vi "$UTIL_Timer.vi"(8 "Auto Reset":bool=TRUE, 9 "Reset":bool, 10 "Time (sec)":dbl=3.0, 11 "Start":bool) -> (0 "Timed Out":bool, 1 "Running":bool, 2 "Numeric 2":dbl, 3 "Elapsed":dbl, 4 "TO Trig":bool, 5 "Is Reset?":bool)   [LabVIEW 2024]
doc: "Uses the second timer to determind when Time (sec) have passed when Start is TRUE. The actual time passes is captured in Lap (sec) \nAutoReset is enabled by default. When enabled, at time out, the values is captured, and the TimeOut set to TRUE for one loop then both are RESET. When not enabled, then a RESET command or another START command are requied to reset both the value and TimeOut Flag.\n\n(The functionality could be expanded to measure elapse time on Mark.)"
panel:
  in  "Init":bool
  out "Boolean":bool=TRUE
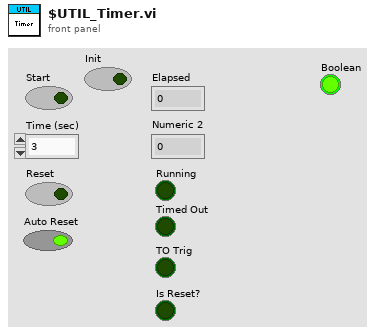
[diagram p1: front panel]
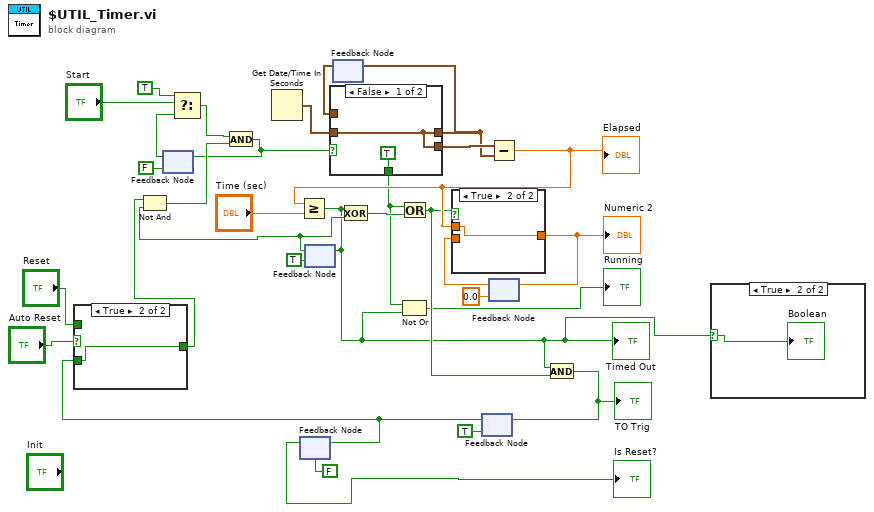
[diagram p0: block diagram]
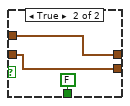
[diagram p5: hidden frame]
diagram:
  n1 = feedback #1(FALSE) -> (w18:bool)
  n2 = Select(t=TRUE, s="Start", f=w18) -> (s? t:f=w16:bool)
  n3 = Get Date/Time In Seconds() -> (seconds since 1Jan1904=w21:timestamp)
  n4 = feedback #2(FALSE) -> (→"Is Reset?":bool)
  n5 = feedback #3(TRUE) -> (w15:bool)
  n6 = feedback #4() -> (w22:timestamp)  [unwired: 1 in]
  n7 = feedback #5(TRUE) -> (w3:bool)
  n8 = case shown="True" "Auto Reset" {
    tunnel: "Reset" -> [w32 _]
    tunnel: [w32 w33] -> w12
    tunnel: w3 -> [_ w33]
    frame False {
    }
    frame True {
    }
  }
  n9 = Not And(1:w15, 2:w12) -> (0:w6:bool)
  n10 = And(x=w16, y=w6) -> (x .and. y?=w4:bool)
  n11 = feedback-in #1(w4) -> ()
  n12 = feedback-in #2(w3) -> ()
  n13 = case shown="False" w4 {
    tunnel: w21 -> [w35 w37]
    tunnel: [w35 w38] -> w23
    tunnel: w22 -> [_ w38]
    tunnel: [w35 w37] -> w24
    tunnel: [TRUE FALSE] -> w8
    frame False {
    }
    frame True {
    }
  }
  n14 = feedback-in #4(w23) -> ()
  n15 = Subtract(x=w24, y=w23) -> (x-y=w29:dbl)
  "Elapsed" <- w29
  n16 = Greater Or Equal?(x=w29, y="Time (sec)") -> (x >= y?=w5:bool)
  "Timed Out" <- w5
  n17 = feedback-in #3(w5) -> ()
  n18 = Exclusive Or(1:w15, 2:w5) -> (0:w30:bool)
  n19 = Not Or(1:w5, 2:w8) -> (0:→"Running":bool)
  n20 = Or(x=w8, y=w30) -> (x .or. y?=w14:bool)
  n21 = feedback #6(0.0) -> (w26:dbl)
  n22 = case shown="True" w14 {
    tunnel: [w39 w40] -> w25
    tunnel: w26 -> [w39 _]
    tunnel: w29 -> [_ w40]
    frame False {
    }
    frame True {
    }
  }
  "Numeric 2" <- w25
  n23 = feedback-in #6(w25) -> ()
  n24 = And(x=w5, y=w14) -> (x .and. y?=w11:bool)
  "TO Trig" <- w11
  n25 = feedback-in #5(w11) -> ()
  n26 = case shown="True" w5 {
    selector: w5 -> [_ w41]
    frame False {
    }
    frame True {
      "Boolean" <- w41
    }
  }
